vi "testing odor and manifold configuration_v4.vi"() -> ()   [LabVIEW 2021]
uses:
  type-defs/odor color (type def).ctl
  type-defs/odor selection (type def).ctl
  type-defs/odor info cluster (type def).ctl
  type-defs/odor description array (type def).ctl
  type-defs/port number (type def).ctl
  type-defs/single port single odor cluster.ctl
  type-defs/manifold selection.ctl
  type-defs/manifold configuration cluster (type def).ctl
  type-defs/manifold configuration cluster array (type def).ctl
  type-defs/odor and manifold config UI states (type def).ctl
  <vilib>/ErrorRing/Error Ring.xnode
  <vilib>/Utility/error.llb/Error Cluster From Error Code.vi
panel:
  in  "generate error":bool
  out "state":T1
  in  "load config":bool
  in  "save config":bool
  out "cycle number":i32
  in  "odor config":T2
  in  "manifold config":T6
  out "error out":errorcluster
  in  "error in (no error)":errorcluster
  in  "Stop":bool
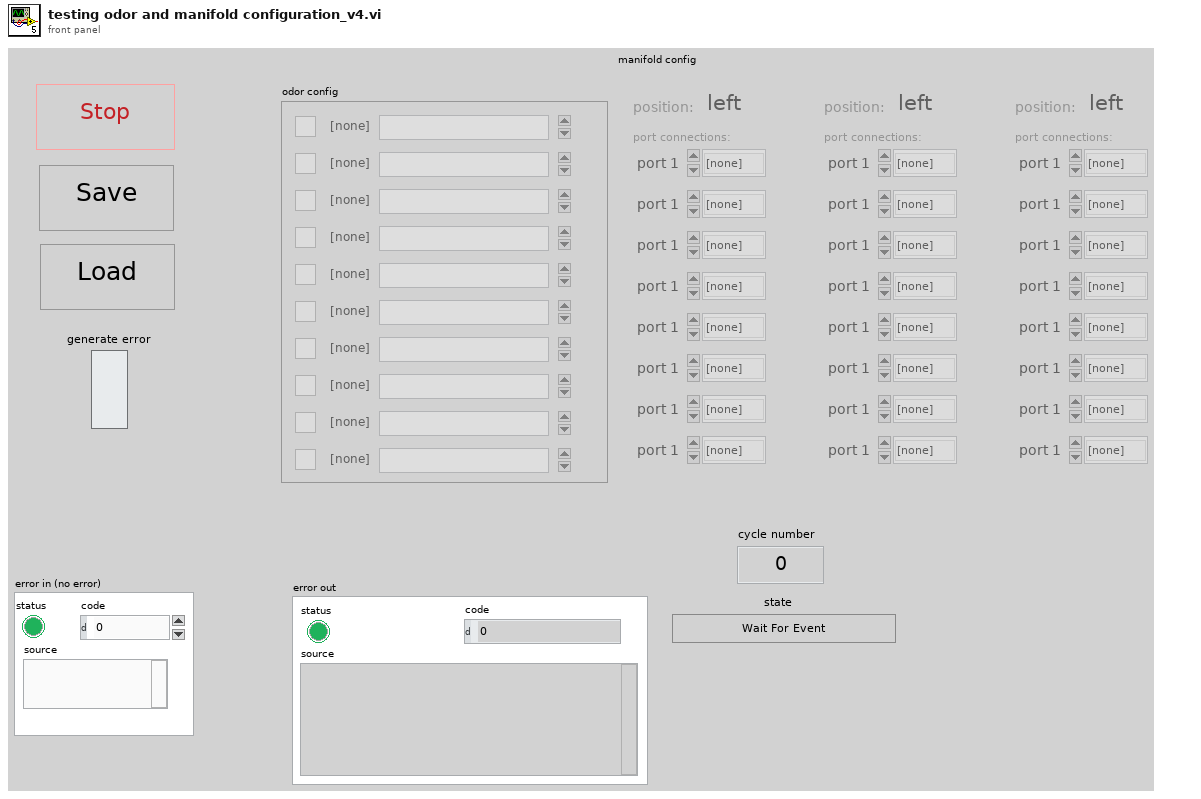
[diagram p1: front panel]
types:
  T1 = typedef "odor and manifold config UI states (type def).ctl" = enum16{"Wait For Event", "Initialize", "Update Odor Config [] Control", "Update Manifold Config [] Control", "Load Config From File", "Handle Errors", "Save Config To File", "Exit"}
  T2 = typedef "odor description array (type def).ctl" = T3[]
  T3 = typedef "odor info cluster (type def).ctl" = cluster{"odor channel":T4, "odor description":string, "odor color":T5, "odor channel active":bool}
  T4 = typedef "odor selection (type def).ctl" = enum16{"[none]", "odor 1", "odor 2", "odor 3", "odor 4", "odor 5", "odor 6", "odor 7", "odor 8", "odor 9", "odor 10"}
  T5 = typedef "odor color (type def).ctl" = u16
  T6 = typedef "manifold configuration cluster array (type def).ctl" = T7[]
  T7 = typedef "manifold configuration cluster (type def).ctl" = cluster{"position:":T8, "port connections:":T9[]}
  T8 = typedef "manifold selection.ctl" = enum16{"left", "middle", "right"}
  T9 = typedef "single port single odor cluster.ctl" = cluster{"port number":T10, "connected odor":T4, "error":bool, "odor color":T5}
  T10 = typedef "port number (type def).ctl" = enum16{"port 1", "port 2", "port 3", "port 4", "port 5", "port 6", "port 7", "port 8"}
  T11 = enum16{"open", "replace", "create", "open or create", "replace or create", "replace or create with confirmation"}
  T12 = enum16{"big-endian, network order", "native, host order", "little-endian"}
  T13 = enum8{"Enabled", "Disabled", "Disabled and Grayed Out"}
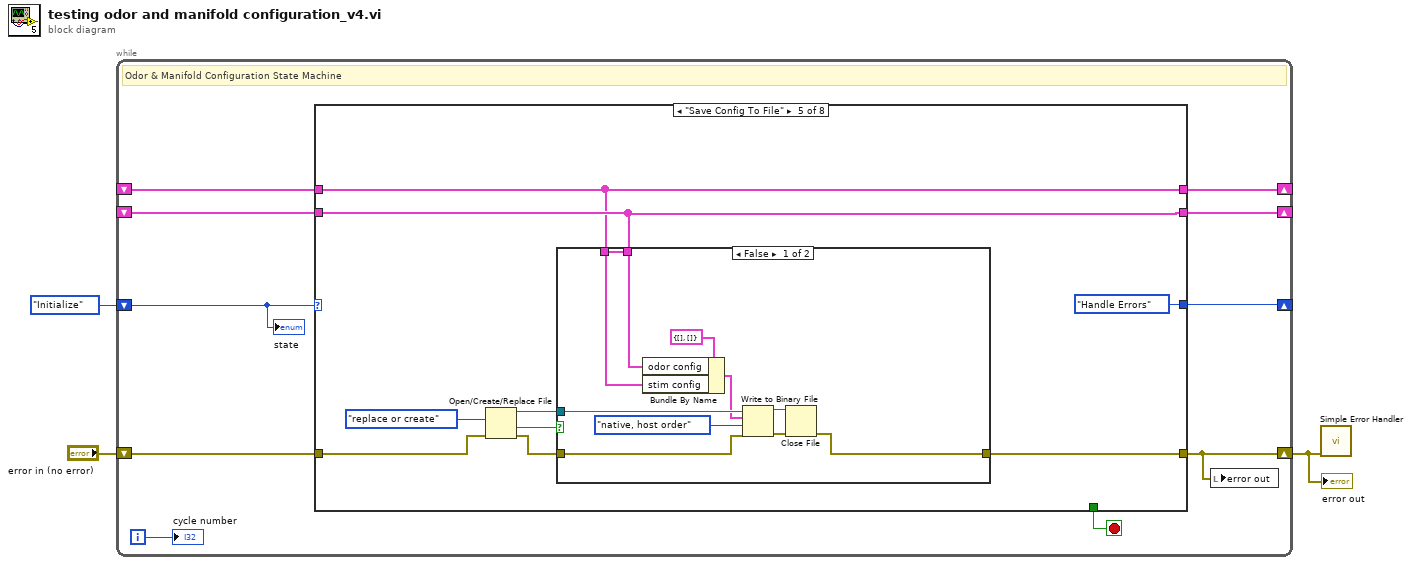
[diagram p0: block diagram]
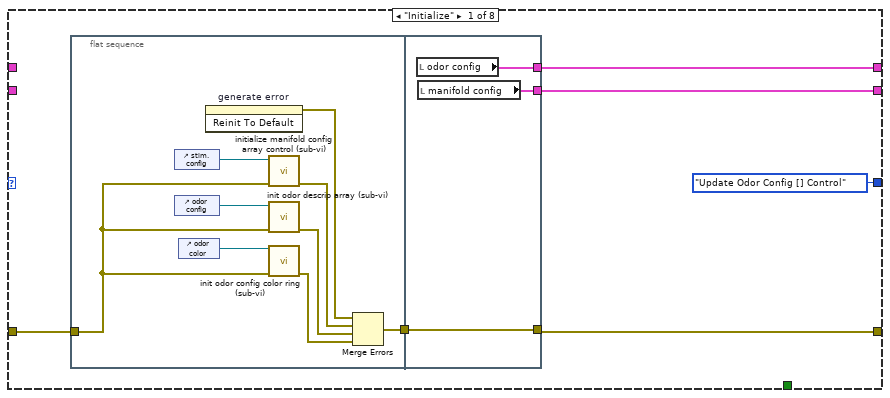
[diagram p2: hidden frame]
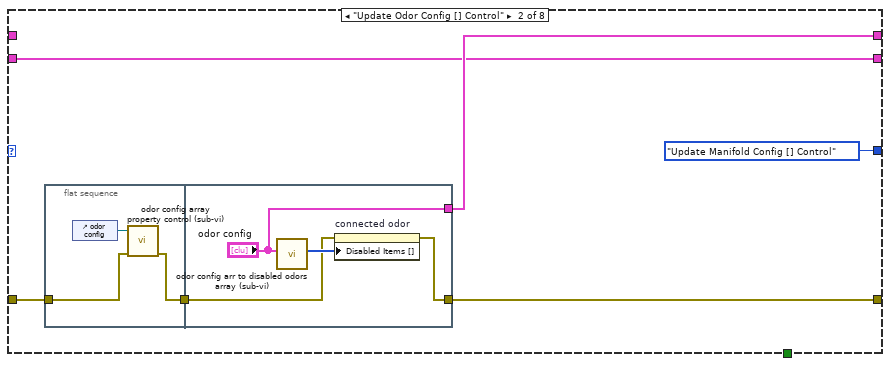
[diagram p3: hidden frame]
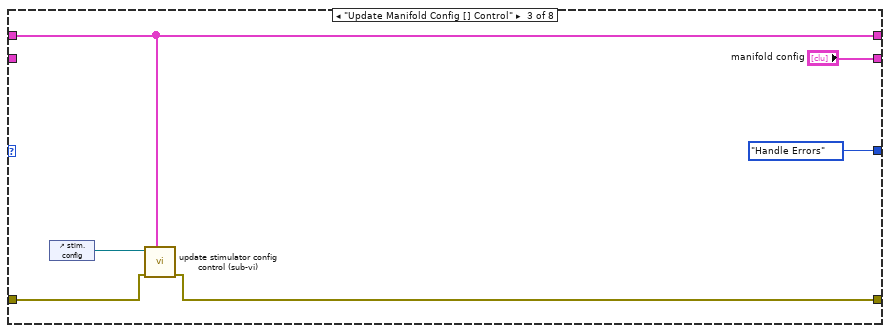
[diagram p4: hidden frame]
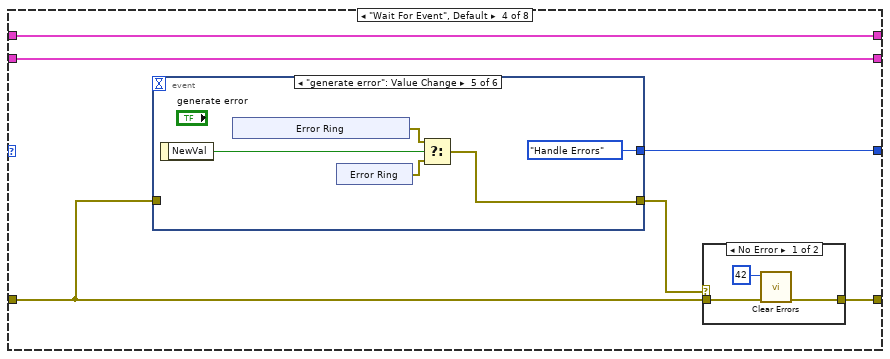
[diagram p5: hidden frame]
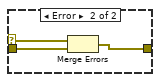
[diagram p6: hidden frame]
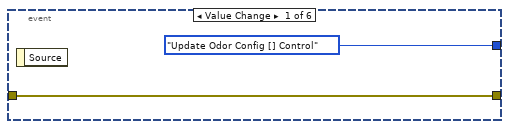
[diagram p7: hidden frame]
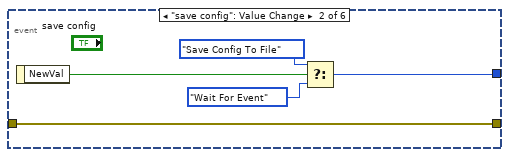
[diagram p8: hidden frame]
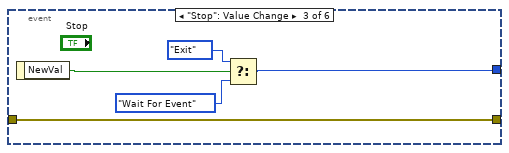
[diagram p9: hidden frame]
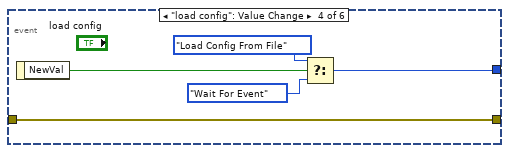
[diagram p10: hidden frame]
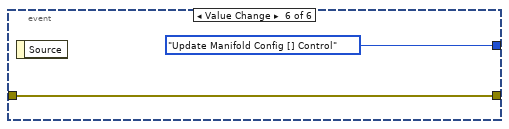
[diagram p11: hidden frame]
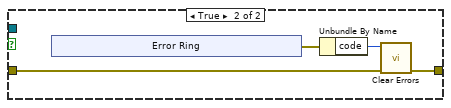
[diagram p12: hidden frame]
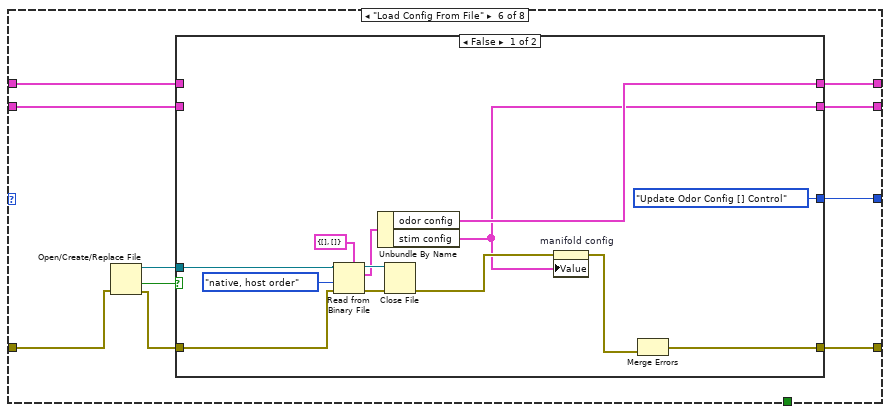
[diagram p13: hidden frame]
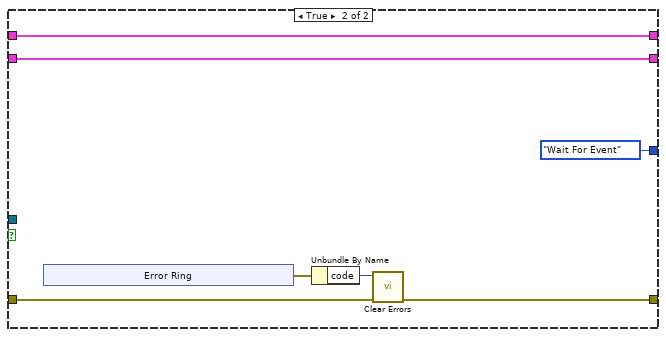
[diagram p14: hidden frame]
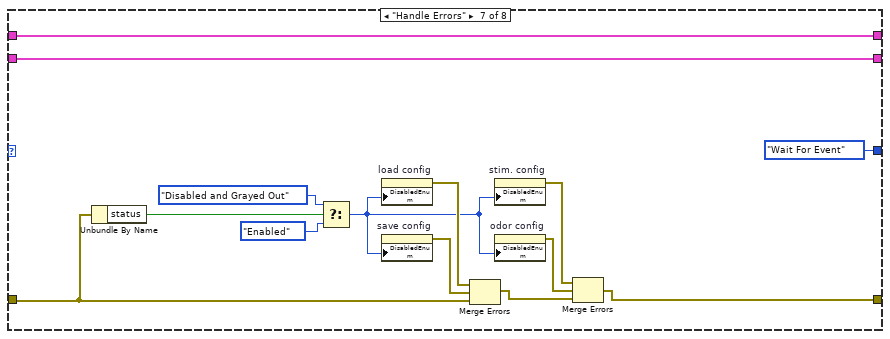
[diagram p15: hidden frame]
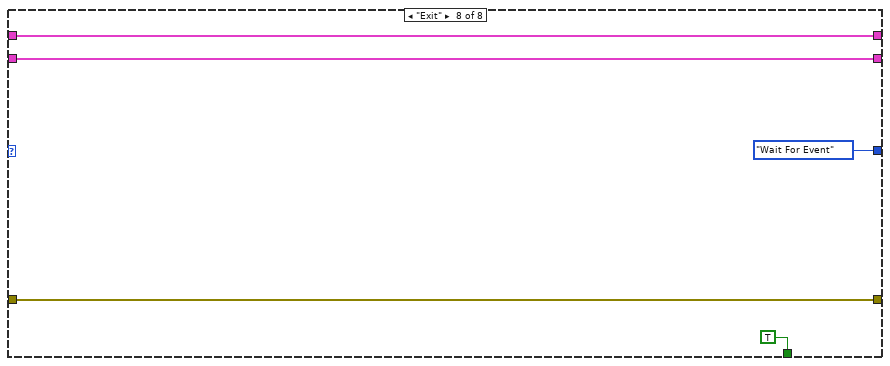
[diagram p16: hidden frame]
diagram:
  n1 = while {
    shift-right: [w4] -> w1
    shift-left: "error in (no error)" -> [w13]
    shift-right: [w12] -> _
    shift-left: _ -> [w11]
    shift-right: [w10] -> _
    shift-left: _ -> [w9]
    shift-right: [w6] -> _
    shift-left: odor_and_manifold_config_UI_states_(type_def)."Initialize" ("Enum") -> [w5]
    i -> [w7]
    stop <- w8 stop-if-true
    # "Odor & Manifold Configuration State Machine"
    n2 = case shown="\"Save Config To File\"" w5 {
      tunnel: w13 -> [w19 w36 w49 w51 w98 w126 w160 w170]
      tunnel: [w18 w35 w48 w52 w95 w125 w156 w170] -> w4
      tunnel: [odor_and_manifold_config_UI_states_(type_def)."Update Odor Config [] Control" ("Enum") odor_and_manifold_config_UI_states_(type_def)."Update Manifold Config [] Control" ("Enum") odor_and_manifold_config_UI_states_(type_def)."Handle Errors" ("Enum") w56 odor_and_manifold_config_UI_states_(type_def)."Handle Errors" ("Enum") w122 odor_and_manifold_config_UI_states_(type_def)."Wait For Event" ("Enum") odor_and_manifold_config_UI_states_(type_def)."Wait For Event" ("Enum")] -> w6
      tunnel: [w14 w34 w45 w55 w93 w120 w166 w171] -> w12
      tunnel: w11 -> [_ _ w45 w55 w93 w121 w166 w171]
      tunnel: [w15 w32 "manifold config" w54 w94 w119 w167 w172] -> w10
      tunnel: w9 -> [_ w32 _ w54 w94 w123 w167 w172]
      tunnel: [_ _ _ _ _ _ _ TRUE] -> w8
      frame "Initialize" {
        n3 = flat-sequence {
          tunnel: w19 -> [w25]
          tunnel: [w24] -> w16
          tunnel: [w31] -> w18
          tunnel: w16 -> [w31]
          tunnel: [w30] -> w15
          tunnel: [w29] -> w14
          frame #0 {
            n4 = control-ref of="stim. config"() -> (w23:refnum<vi>)
            n5 = control-ref of="odor config"() -> (w22:refnum<vi>)
            n6 = control-ref of="odor color"() -> (w21:refnum<vi>)
            n7 = invoke on="generate error" class="Bool (strict)" method="Reinit To Default"() -> (error out=w20:errorcluster)  [unwired: 3 in, 2 out]
            n8 = call "initialize manifold config array control (sub-vi).vi"("error in (no error)"=w25, "stimulator config array refnum"=w23) -> ("error out"=w28:errorcluster)  [unwired: 8 in, 1 out]
            n9 = call "init odor descrip array (sub-vi).vi"("error in (no error)"=w25, "array refnum"=w22) -> ("error out"=w27:errorcluster)  [unwired: 8 in, 1 out]
            n10 = call "init odor config color ring (sub-vi).vi"("error in (no error)"=w25, "ring refnum"=w21) -> ("error out"=w26:errorcluster)  [unwired: 8 in, 1 out]
            n11 = Merge Errors(w20, w28, w27, w26) -> (w24:errorcluster)
          }
          frame #1 {
            n12 = local read "odor config"() -> (w29:T2)
            n13 = local read "manifold config"() -> (w30:T6)
          }
        }
      }
      frame "Update Odor Config [] Control" {
        n14 = flat-sequence {
          tunnel: [w40] -> w37
          tunnel: w36 -> [w39]
          tunnel: w37 -> [w43]
          tunnel: [w42] -> w35
          tunnel: ["odor config"] -> w34
          frame #0 {
            n15 = control-ref of="odor config"() -> (w38:refnum<vi>)
            n16 = call "odor config array property control (sub-vi).vi"("error in (no error)"=w39, "odor config array refnum"=w38) -> ("error out"=w40:errorcluster)  [unwired: 8 in, 1 out]
          }
          frame #1 {
            n17 = call "odor config arr to disabled odors array (sub-vi).vi"("odor descriptions"="odor config") -> ("Disabled Items []"=w44:i32[])  [unwired: 10 in]
            n18 = property on="connected odor" class="Enum (strict)"(error in=w43, "Disabled Items []"=w44) -> (error out=w42:errorcluster)  [unwired: 1 in, 1 out]
          }
        }
      }
      frame "Update Manifold Config [] Control" {
        n19 = control-ref of="stim. config"() -> (w50:refnum<vi>)
        n20 = call "update stimulator config control (sub-vi).vi"("odor config array"=w45, "error in (no error)"=w49, "manifold config array refnum"=w50) -> ("error out"=w48:errorcluster)  [unwired: 6 in, 2 out]
      }
      frame "Wait For Event", Default {
        n21 = event shown="[4] \"generate error\": Value Change" {
          selector: _ -> [_ _ _ _ _ _]
          dyn-events: _ -> [_ _ _ _ _ _]
          timeout: _ -> [_ _ _ _ _ _]
          tunnel: [odor_and_manifold_config_UI_states_(type_def)."Update Odor Config [] Control" ("Enum") w66 w72 w76 odor_and_manifold_config_UI_states_(type_def)."Handle Errors" ("Enum") odor_and_manifold_config_UI_states_(type_def)."Update Manifold Config [] Control" ("Enum")] -> w56
          tunnel: [w63 w65 w70 w75 w80 w90] -> w53
          tunnel: w51 -> [w63 w65 w70 w75 _ w90]
          event Value Change {
            n22 = event-data() -> ()  [unwired: 1 in, 1 out]
          }
          event "save config": Value Change {
            n23 = event-data() -> ("NewVal"=w69:bool)  [unwired: 1 in]
            n24 = Select(t=odor_and_manifold_config_UI_states_(type_def)."Save Config To File", s=w69, f=odor_and_manifold_config_UI_states_(type_def)."Wait For Event" ("Enum")) -> (s? t:f=w66:T1)
          }
          event "Stop": Value Change {
            n25 = event-data() -> ("NewVal"=w74:bool)  [unwired: 1 in]
            n26 = Select(t=odor_and_manifold_config_UI_states_(type_def)."Exit", s=w74, f=odor_and_manifold_config_UI_states_(type_def)."Wait For Event" ("Enum")) -> (s? t:f=w72:T1)
          }
          event "load config": Value Change {
            n27 = event-data() -> ("NewVal"=w79:bool)  [unwired: 1 in]
            n28 = Select(t=odor_and_manifold_config_UI_states_(type_def)."Load Config From File", s=w79, f=odor_and_manifold_config_UI_states_(type_def)."Wait For Event" ("Enum")) -> (s? t:f=w76:T1)
          }
          event "generate error": Value Change {
            n29 = event-data() -> ("NewVal"=w84:bool)  [unwired: 1 in]
            n30 = xnode "Error Ring"() -> ("error out"=w82:errorcluster)
            n31 = xnode "Error Ring"() -> ("error out"=w83:errorcluster)
            n32 = Select(t=w82, s=w84, f=w83) -> (s? t:f=w80:errorcluster)
          }
          event Value Change {
            n33 = event-data() -> ()  [unwired: 1 in, 1 out]
          }
        }
        n34 = case shown="No Error" w53 {
          selector: w53 -> [_ w62]
          tunnel: [w58 w60] -> w52
          tunnel: w51 -> [w59 w61]
          frame No Error {
            n35 = call <vilib>:"Clear Errors.vi"("error in (no error)"=w59, "specific error code to clear (0: all)"=42) -> ("error out"=w58:errorcluster)  [unwired: 4 in, 1 out]
          }
          frame Error {
            n36 = Merge Errors(w62, w61) -> (w60:errorcluster)
          }
        }
      }
      frame "Save Config To File" {
        n37 = Open/Create/Replace File(error in=w98, operation (0:open)=T11."replace or create") -> (refnum out=w100:refnum<file>, cancelled=w96:bool, error out=w97:errorcluster)  [unwired: 4 in]
        n38 = case shown="False" w96 {
          tunnel: w100 -> [w109 _]
          tunnel: w97 -> [w104 w112]
          tunnel: [w103 w111] -> w95
          tunnel: w93 -> [w102 _]
          tunnel: w94 -> [w101 _]
          frame False {
            n39 = Bundle By Name(cluster=cluster{"stim config":T6, "odor config":T2} {"stim config"=[], "odor config"=[]} ("Cluster"), "odor config"=w102, "stim config"=w101) -> (w108:cluster{"stim config":T6, "odor config":T2})
            n40 = Write to Binary File(file (use dialog)=w109, data=w108, error in=w104, 9:T12."native, host order" ("byte order (0:big-endian, network order)")) -> (refnum out=w106:refnum<file>, error out=w107:errorcluster)  [unwired: 2 in, 1 out]
            n41 = Close File(refnum=w106, error in=w107) -> (error out=w103:errorcluster)  [unwired: 1 out]
          }
          frame True {
            n42 = xnode "Error Ring"() -> ("error out"=w114:errorcluster)
            n43 = Unbundle By Name(w114) -> ("code"=w113:i32)
            n44 = call <vilib>:"Clear Errors.vi"("error in (no error)"=w112, "specific error code to clear (0: all)"=w113) -> ("error out"=w111:errorcluster)  [unwired: 4 in, 1 out]
          }
        }
      }
      frame "Load Config From File" {
        n45 = Open/Create/Replace File(error in=w126) -> (refnum out=w127:refnum<file>, cancelled=w124:bool, error out=w128:errorcluster)  [unwired: 5 in]
        n46 = case shown="False" w124 {
          tunnel: w128 -> [w142 w146]
          tunnel: w127 -> [w141 _]
          tunnel: [w133 w145] -> w125
          tunnel: w123 -> [_ w147]
          tunnel: w121 -> [_ w148]
          tunnel: [odor_and_manifold_config_UI_states_(type_def)."Update Odor Config [] Control" ("Enum") odor_and_manifold_config_UI_states_(type_def)."Wait For Event" ("Enum")] -> w122
          tunnel: [w130 w148] -> w120
          tunnel: [w129 w147] -> w119
          frame False {
            n47 = Read from Binary File(5:cluster{"stim config":T6, "odor config":T2} {"stim config"=[], "odor config"=[]} ("Cluster"), 8:w142, 9:T12."native, host order" ("byte order (0:big-endian, network order)"), 11:w141) -> (0:w140:errorcluster, 2:w137:cluster{"stim config":T6, "odor config":T2}, 3:w139:refnum<file>)  [unwired: 2 in, 1 out]
            n48 = Unbundle By Name(w137) -> ("odor config"=w130:T2, "stim config"=w129:T6)
            n49 = Close File(refnum=w139, error in=w140) -> (error out=w132:errorcluster)  [unwired: 1 out]
            n50 = property on="manifold config" class="Arr (strict)"(error in=w132, "Value"=w129) -> (error out=w135:errorcluster)  [unwired: 1 in, 1 out]
            n51 = Merge Errors(w135) -> (w133:errorcluster, w136:errorcluster)
          }
          frame True {
            n52 = xnode "Error Ring"() -> ("error out"=w144:errorcluster)
            n53 = Unbundle By Name(w144) -> ("code"=w143:i32)
            n54 = call <vilib>:"Clear Errors.vi"("error in (no error)"=w146, "specific error code to clear (0: all)"=w143) -> ("error out"=w145:errorcluster)  [unwired: 4 in, 1 out]
          }
        }
      }
      frame "Handle Errors" {
        n55 = Unbundle By Name(w160) -> ("status"=w164:bool)
        n56 = Select(t=T13."Disabled and Grayed Out", s=w164, f=T13."Enabled" ("Disabled")) -> (s? t:f=w157:T13)
        n57 = property on="load config" class="Bool"("DisabledEnum"=w157) -> (error out=w161:errorcluster)  [unwired: 2 in, 1 out]
        n58 = property on="save config" class="Bool"("DisabledEnum"=w157) -> (error out=w162:errorcluster)  [unwired: 2 in, 1 out]
        n59 = Merge Errors(w161, w162, w160) -> (w159:errorcluster)
        n60 = property on="stim. config" class="Arr (strict)"("DisabledEnum"=w157) -> (error out=w154:errorcluster)  [unwired: 2 in, 1 out]
        n61 = property on="odor config" class="Arr (strict)"("DisabledEnum"=w157) -> (error out=w155:errorcluster)  [unwired: 2 in, 1 out]
        n62 = Merge Errors(w154, w155, w159) -> (w156:errorcluster)
      }
      frame "Exit" {
      }
    }
    n63 = local write "error out"(w4) -> ()
    "state" <- w5
    "cycle number" <- w7
  }
  "error out" <- w1
  n64 = call <vilib>:"Simple Error Handler.vi"("error in (no error)"=w1) -> ()  [unwired: 4 in, 5 out]
